vi "Server2.vi"() -> ()   [LabVIEW 2020]
panel:
  in  "stop":bool
  # "VI Server"
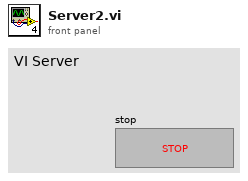
[diagram p1: front panel]
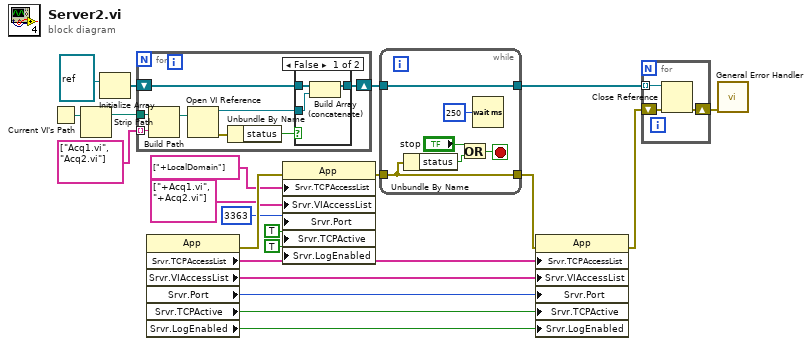
[diagram p0: block diagram]
diagram:
  n1 = Current VI's Path() -> (path=w10:path)
  n2 = Strip Path(path=w10) -> (stripped path=w9:path)  [unwired: 1 out]
  n3 = Initialize Array(refnum<vi> refnum) -> (w14:refnum<vi>[])  [unwired: 1 in]
  n4 = for {
    tunnel: string[] ["Acq1.vi", "Acq2.vi"] ("Server:VI Access List") -> [w29] mode=indexing
    shift-right: [w24] -> w2
    shift-left: w14 -> [w25]
    tunnel: w9 -> [w23]
    n5 = Build Path(base path=w23, name or relative path=w29) -> (appended path=w30:path)
    n6 = Open VI Reference(vi path=w30) -> (vi reference=w26:refnum<vi>, error out=w27:errorcluster)  [unwired: 5 in]
    n7 = Unbundle By Name(w27) -> ("status"=w28:bool)
    n8 = case shown="False" w28 {
      tunnel: w26 -> [w31 _]
      tunnel: w25 -> [w33 w34]
      tunnel: [w32 w34] -> w24
      frame False {
        n9 = Build Array (concatenate)(w33, w31) -> (w32:refnum<vi>[])
      }
      frame True {
      }
    }
  }
  n10 = property class="App"() -> (error out=w22:errorcluster, "Srvr.TCPAccessList"=w19:string[], "Srvr.VIAccessList"=w18:string[], "Srvr.Port"=w17:u32, "Srvr.TCPActive"=w16:bool, "Srvr.LogEnabled"=w15:bool)  [unwired: 2 in, 1 out]
  n11 = property class="App"(error in=w22, "Srvr.TCPAccessList"=string[] ["+LocalDomain"] ("Server:TCP/IP Access List"), "Srvr.VIAccessList"=string[] ["+Acq1.vi", "+Acq2.vi"] ("Server:VI Access List"), "Srvr.Port"=u32 3363 ("Server:Port"), "Srvr.TCPActive"=TRUE ("Server:TCP Listener Active"), "Srvr.LogEnabled"=TRUE ("Server:Logging Enabled")) -> (error out=w21:errorcluster)  [unwired: 1 in, 1 out]
  n12 = while {
    tunnel: w21 -> [w38]
    tunnel: [w38] -> w20
    tunnel: w2 -> [w37]
    tunnel: [w37] -> w1
    stop <- w39 stop-if-true
    n13 = Unbundle By Name(w38) -> ("status"=w36:bool)
    n14 = Or(x="stop", y=w36) -> (x .or. y?=w39:bool)
    n15 = Wait (ms)(milliseconds to wait=u32 250) -> ()  [unwired: 1 out]
  }
  n16 = property class="App"(error in=w20, "Srvr.TCPAccessList"=w19, "Srvr.VIAccessList"=w18, "Srvr.Port"=w17, "Srvr.TCPActive"=w16, "Srvr.LogEnabled"=w15) -> (error out=w11:errorcluster)  [unwired: 1 in, 1 out]
  n17 = for {
    shift-right: [w42] -> w12
    shift-left: w11 -> [w43]
    tunnel: w1 -> [w41] mode=indexing
    n18 = Close Reference(reference=w41, error in (no error)=w43) -> (error out=w42:errorcluster)
  }
  n19 = call <vilib>:"General Error Handler.vi"("error in (no error)"=w12) -> ()  [unwired: 10 in, 5 out]
